vi "ToDatagram.vi"(8 "error in (no error)":errorcluster, 10 "messageID":u16, 11 "DisconnectMqttMsg in":refnum<class "DisconnectMqttMsg.lvclass">) -> (0 "error out":errorcluster, 2 "Datagram":u8[](array[numeric]), 3 "DisconnectMqttMsg out":refnum<class "DisconnectMqttMsg.lvclass">)   [LabVIEW 2020, in "DisconnectMqttMsg.lvclass"]
uses:
  DisconnectMqttMsg.lvclass
  mqttTypedef/QosLevel.ctl
  mqttTypedef/MessageType.ctl
  BaseMqttMsg.lvclass
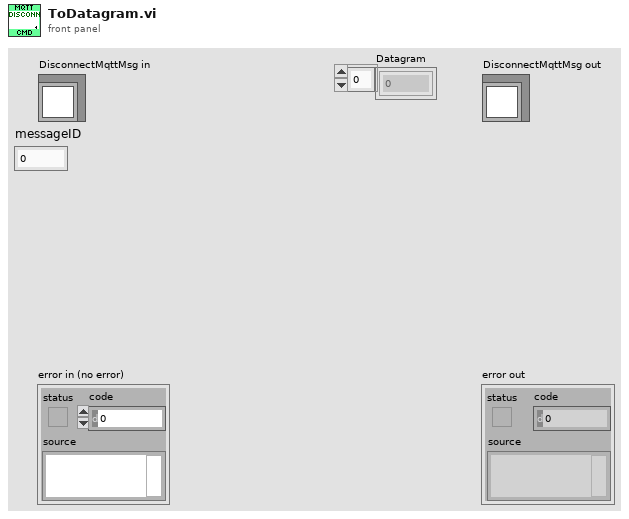
[diagram p1: front panel]
types:
  T1 = typedef "BaseMqttMsg.lvclass/MessageType.ctl" = enum32{"Reserved", "CONNECT", "CONNACK", "PUBLISH", "PUBACK", "PUBREC", "PUBREL", "PUBCOMP", "SUBSCRIBE", "SUBACK", "UNSUBSCRIBE", "UNSUBACK", "PINGREQ", "PINGRESP", "DISCONNECT", "Reserved2"}
  T2 = typedef "BaseMqttMsg.lvclass/QosLevel.ctl" = enum8{"At most once", "At least once", "Exactly once", "Reserved"}
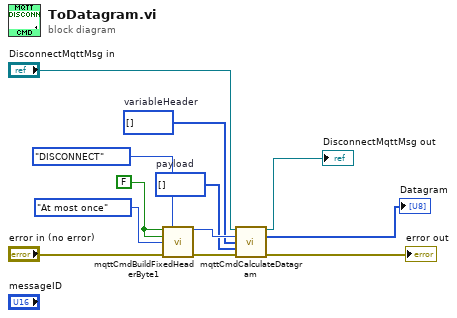
[diagram p0: block diagram]
diagram:
  w7 = u8[] []  # payload
  w8 = u8[] []  # variableHeader
  w11 = FALSE
  n1 = call "mqttCmdBuildFixedHeaderByte1.vi"("retain(F)"=w11, "MessageType"=MessageType."DISCONNECT", "duplicate(F)"=w11, "QoS (At most once)"=QosLevel."At most once", "error in (no error)"="error in (no error)") -> ("byte1"=w9:u8, "error out"=w6:errorcluster)  [unwired: 9 in]
  n2 = call-dynamic "mqttCmdCalculateDatagram.vi"("mqttCmd in"="DisconnectMqttMsg in", "FixedHeaderByte1"=w9, "variableHeader"=w8, "payload"=w7, "error in (no error)"=w6) -> ("mqttCmd out"=→"DisconnectMqttMsg out":refnum<class "DisconnectMqttMsg.lvclass">, "Datagram"=→"Datagram":u8[], "error out"=→"error out":errorcluster)  [unwired: 8 in]
